vi "Execute.vi"(8 "error in (no error)":errorcluster, 11 "Node in":refnum<class "Set Boolean.lvclass">) -> (0 "error out":errorcluster, 1 "Status":T1, 3 "Node out":refnum<class "Set Boolean.lvclass">)   [LabVIEW 2021, in "BT.lvlib" / "Set Boolean.lvclass"]
uses:
  Set Boolean.lvclass
  C:/Users/Tim/Documents/GitHub/LV_Behaviour_Tree/Source/Support/Nodes/Leaves/abs_Type Leaf/abs_Type Leaf.lvclass
  abs_Node/Status.ctl
  <vilib>/TSA/Abstract Data Classes/Abs_Types/Boolean/Abs_Boolean.lvclass
  C:/Program Files (x86)/National Instruments/LabVIEW 2021/vi.lib/TSA/Abstract Data Classes/Abs_Types/Type/Abs_Type.lvclass
  abs_Type Leaf/abs_Type Leaf.lvclass/abs_Type Leaf.ctl
  Set Boolean.lvclass/Set Boolean.ctl
  abs_Type Leaf/Properties/Read Value Class.vi
  Properties/Read Boolean.vi
  abs_Type Leaf/Properties/Write Value Class.vi
  abs_Type Leaf/abs_Type Leaf.lvclass
  <vilib>/TSA/Abstract Data Classes/Abs_Types/Type/Abs_Type.lvclass
  abs_Node/bt_Node.lvclass
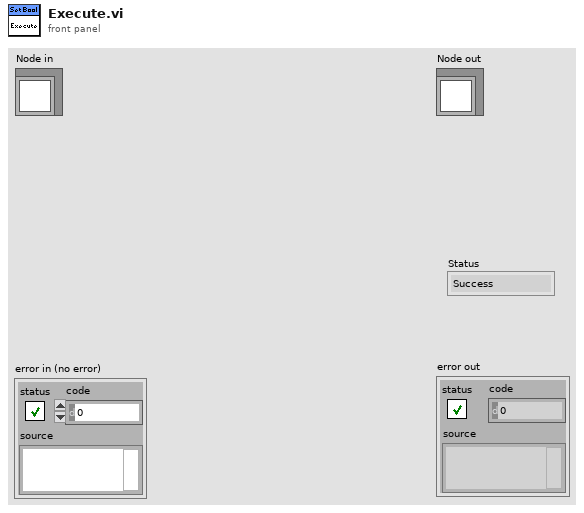
[diagram p1: front panel]
types:
  T1 = typedef "BT.lvlib/bt_Node.lvclass/Status.ctl" = enum16{"Success", "Failure", "Running"}
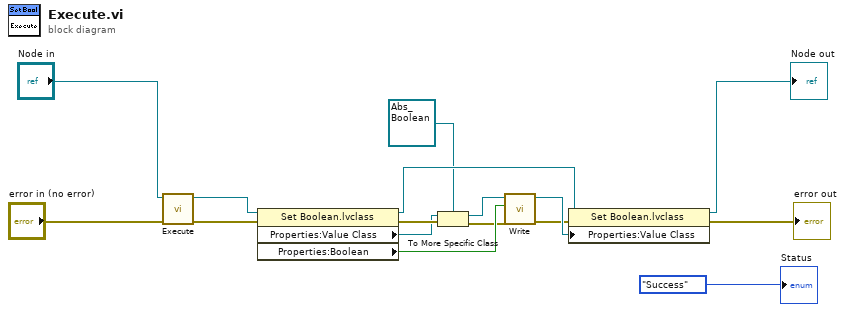
[diagram p0: block diagram]
diagram:
  n1 = call-parent "Execute.vi"("error in (no error)"="error in (no error)", "Node in"="Node in") -> ("error out"=w11:errorcluster, "Node out"=w10:refnum<class "Set Boolean.lvclass">)  [unwired: 7 in, 1 out]
  n2 = property class="Set Boolean.lvclass"(reference=w10, error in=w11) -> (reference out=w9:refnum<class "Set Boolean.lvclass">, error out=w5:errorcluster, "Properties:Value Class"=w4:refnum<class "Abs_Type.lvclass">, "Properties:Boolean"=w6:bool)
  n3 = To More Specific Class(target class=refnum<class "Abs_Boolean.lvclass"> refnum ("Boolean in"), reference=w4, error in=w5) -> (specific class reference=w1:refnum<class "Abs_Boolean.lvclass">, error out=w3:errorcluster)
  n4 = call-dynamic "Write.vi"("error in (no error)"=w3, "Boolean"=w6, "Boolean in"=w1) -> ("error out"=w7:errorcluster, "Boolean out"=w8:refnum<class "Abs_Boolean.lvclass">)  [unwired: 7 in]
  n5 = property class="Set Boolean.lvclass"(reference=w9, error in=w7, "Properties:Value Class"=w8) -> (reference out=→"Node out":refnum<class "Set Boolean.lvclass">, error out=→"error out":errorcluster)
  "Status" <- Status."Success" ("Status")
